vi "Read Step Context.vi"(8 "error in (no error)":errorcluster, 11 "Execution in":refnum<class "Execution.lvclass">) -> (0 "error out":errorcluster, 2 "Step Context":T1={"StepIndex"=0, "Step"=refnum, "StartTime"=timestamp(0 s since 1904-01-01), "EndTime"=timestamp(0 s since 1904-01-01), "Result"=enum."Error", "Error Info"="", "Output Values"=[]}, 3 "Execution out":refnum<class "Execution.lvclass">)   [LabVIEW 2015, in "Execution.lvclass"]
uses:
  Execution.lvclass
  STEP_CONTEXT.ctl
  Step.lvclass
  Step/STEP_STATUS.ctl
  Execution.lvclass/Execution.ctl
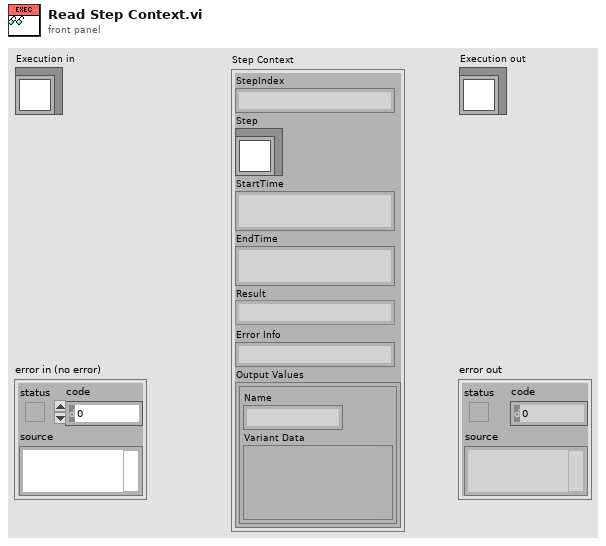
[diagram p1: front panel]
types:
  T1 = typedef "Execution.lvclass/STEP_CONTEXT.ctl" = cluster{"StepIndex":u32, "Step":refnum<class "Step.lvclass">, "StartTime":timestamp, "EndTime":timestamp, "Result":T2, "Error Info":string, "Output Values":cluster{"Name":string, "Variant Data":variant}[]}
  T2 = typedef "Step.lvclass/STEP_STATUS.ctl" = enum16{"Skipped", "Done", "Passed", "Failed", "Error"}
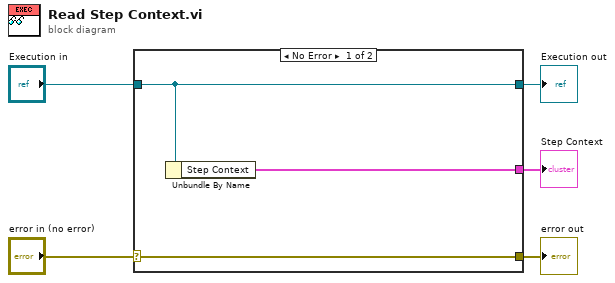
[diagram p0: block diagram]
diagram:
  n1 = case shown="No Error" "error in (no error)" {
    selector: "error in (no error)" -> [w8 w9]
    tunnel: [w8 w9] -> w4
    tunnel: [w7 w10] -> w2
    tunnel: "Execution in" -> [w7 w10]
    tunnel: [w6 _] -> w1
    frame No Error {
      n2 = Unbundle By Name(w7) -> ("Step Context"=w6:T1)
    }
    frame Error {
    }
  }
  "error out" <- w4
  "Execution out" <- w2
  "Step Context" <- w1
